vi "fitting on a circle.vi"(4 "Y":dbl[](array[numeric]) format="%.2f", 5 "X":dbl[](array[numeric]) format="%.2f") -> (0 "error":i32, 1 "r":dbl format="%.2f", 2 "x0, y0":dbl[](array[numeric]) format="%.2f")   [LabVIEW 2020]
uses:
  <vilib>/Analysis/baseanly.llb/Mean (DBL).vi
  <vilib>/Analysis/7linalg.llb/Solve Linear Equations (single right hand).vi
  <vilib>/Analysis/baseanly.llb/Solve Linear Equations By Cholesky.vi
  <vilib>/Analysis/baseanly.llb/Real Matrix to Compact Array.vi
  <vilib>/Analysis/baseanly.llb/Real Compact Tri-Matrix Linear Eqs.vi
  <vilib>/Analysis/7linalg.llb/Solve Linear Eqs (General).vi
  <vilib>/Analysis/7linalg.llb/Solve Linear Eqs (Gen, single right hand).vi
  <vilib>/Analysis/NI_AALBase.lvlib
  <vilib>/Analysis/NI_AALPro.lvlib
panel:
  # "Example:\n\n X: data points\n Y: data points"
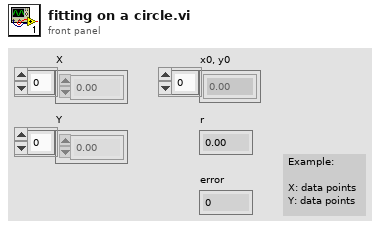
[diagram p1: front panel]
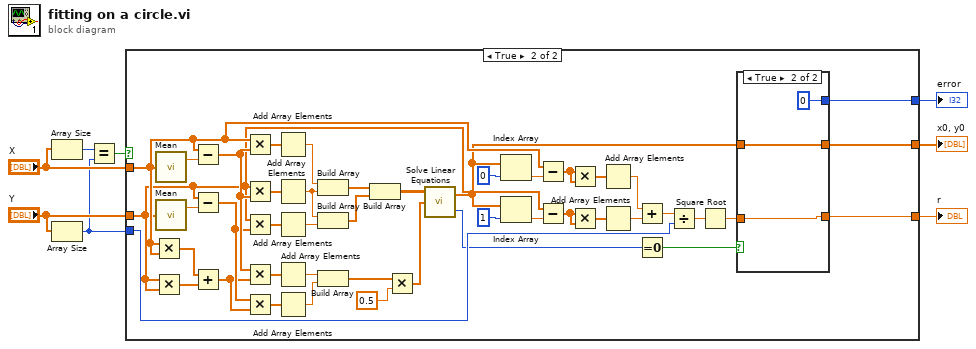
[diagram p0: block diagram]
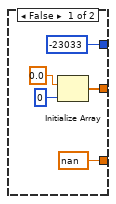
[diagram p2: hidden frame]
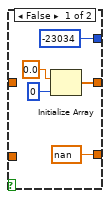
[diagram p3: hidden frame]
diagram:
  n1 = Array Size(array="X") -> (size(s)=w8:i32)
  n2 = Array Size(array="Y") -> (size(s)=w4:i32)
  n3 = Equal?(x=w8, y=w4) -> (x = y?=w7:bool)
  n4 = case shown="True" w7 {
    tunnel: "X" -> [_ w32]
    tunnel: "Y" -> [_ w26]
    tunnel: w4 -> [_ w23]
    tunnel: [-23033 w18] -> w3
    tunnel: [nan w17] -> w2
    tunnel: [w11 w15] -> w1
    frame False {
      n5 = Initialize Array(0.0, 0) -> (w11:dbl[])
    }
    frame True {
      n6 = Multiply(x=w32, y=w32) -> (x*y=w56:dbl[])
      n7 = Multiply(x=w26, y=w26) -> (x*y=w55:dbl[])
      n8 = call-poly <vilib>:"Mean.vi"("X"=w32) -> ("mean"=w58:dbl)  [unwired: 1 out]
      n9 = call-poly <vilib>:"Mean.vi"("X"=w26) -> ("mean"=w57:dbl)  [unwired: 1 out]
      n10 = Subtract(x=w32, y=w58) -> (x-y=w45:dbl[])
      n11 = Subtract(x=w26, y=w57) -> (x-y=w43:dbl[])
      n12 = Add(x=w56, y=w55) -> (x+y=w42:dbl[])
      n13 = Multiply(x=w32, y=w45) -> (x*y=w54:dbl[])
      n14 = Multiply(x=w26, y=w45) -> (x*y=w53:dbl[])
      n15 = Multiply(x=w26, y=w43) -> (x*y=w52:dbl[])
      n16 = Multiply(x=w45, y=w42) -> (x*y=w46:dbl[])
      n17 = Multiply(x=w43, y=w42) -> (x*y=w44:dbl[])
      n18 = Add Array Elements(numeric array=w54) -> (sum=w51:dbl)
      n19 = Add Array Elements(numeric array=w53) -> (sum=w49:dbl)
      n20 = Add Array Elements(numeric array=w52) -> (sum=w50:dbl)
      n21 = Add Array Elements(numeric array=w46) -> (sum=w41:dbl)
      n22 = Add Array Elements(numeric array=w44) -> (sum=w40:dbl)
      n23 = Build Array(w51, w49) -> (w48:dbl[])
      n24 = Build Array(w49, w50) -> (w47:dbl[])
      n25 = Build Array(w41, w40) -> (w38:dbl[])
      n26 = Build Array(w48, w47) -> (w39:dbl[][])
      n27 = Multiply(x=w38, y=0.5) -> (x*y=w36:dbl[])
      n28 = call-poly <vilib>:"Solve Linear Equations.vi"("Known Vector"=w36, "Input Matrix"=w39) -> ("error"=w20:i32, "Solution Vector"=w14:dbl[])  [unwired: 1 in]
      n29 = Index Array(array=w14, index=0) -> (element=w31:dbl)
      n30 = Index Array(array=w14, index=1) -> (element=w27:dbl)
      n31 = Subtract(x=w32, y=w31) -> (x-y=w30:dbl[])
      n32 = Subtract(x=w26, y=w27) -> (x-y=w29:dbl[])
      n33 = Multiply(x=w30, y=w30) -> (x*y=w35:dbl[])
      n34 = Multiply(x=w29, y=w29) -> (x*y=w28:dbl[])
      n35 = Add Array Elements(numeric array=w35) -> (sum=w25:dbl)
      n36 = Add Array Elements(numeric array=w28) -> (sum=w24:dbl)
      n37 = Add(x=w25, y=w24) -> (x+y=w22:dbl)
      n38 = Equal To 0?(x=w20) -> (x = 0?=w19:bool)
      n39 = Divide(x=w22, y=w23) -> (x/y=w21:dbl)
      n40 = Square Root(x=w21) -> (sqrt(x)=w16:dbl)
      n41 = case shown="True" w19 {
        tunnel: [-23034 0] -> w18
        tunnel: [nan w65] -> w17
        tunnel: w16 -> [_ w65]
        tunnel: [w59 w64] -> w15
        tunnel: w14 -> [_ w64]
        frame False {
          n42 = Initialize Array(0.0, 0) -> (w59:dbl[])
        }
        frame True {
        }
      }
    }
  }
  "x0, y0" <- w1
  "error" <- w3
  "r" <- w2
